vi "hpcnc visa write read.vi"(8 "error in (no error)":errorcluster, 10 "Send data":string, 11 "CNC COM in":refnum<visa-resource-name>) -> (0 "error out":errorcluster, 1 "Receive buffer":string, 2 "Receive count":u32, 3 "CNC COM out":refnum<visa-resource-name>)   [LabVIEW 2014, in "HPCNC.lvlib"]
uses:
  HPCNC.lvlib
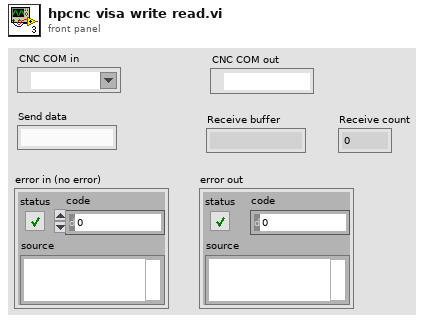
[diagram p1: front panel]
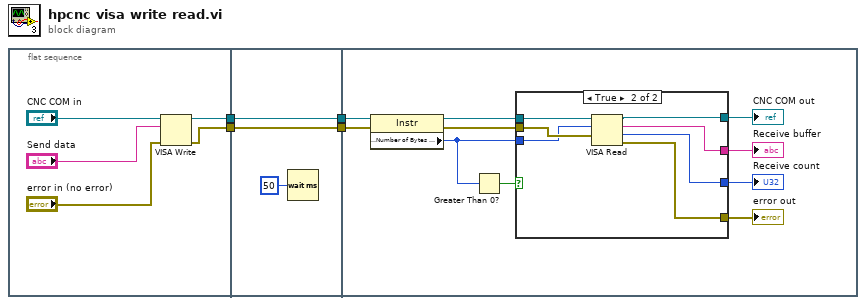
[diagram p0: block diagram]
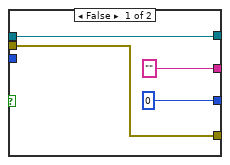
[diagram p2: hidden frame]
diagram:
  n1 = flat-sequence {
    tunnel: [w6] -> w3
    tunnel: [w5] -> w1
    tunnel: [w11] -> w4
    tunnel: w3 -> [w11]
    tunnel: [w10] -> w2
    tunnel: w1 -> [w10]
    tunnel: w4 -> [w14]
    tunnel: w2 -> [w13]
    frame #0 {
      n2 = VISA Write(VISA resource name="CNC COM in", write buffer="Send data", error in (no error)="error in (no error)") -> (VISA resource name out=w6:refnum<visa-resource-name>, error out=w5:errorcluster)  [unwired: 1 out]
    }
    frame #1 {
      n3 = Wait (ms)(milliseconds to wait=u32 50) -> ()  [unwired: 1 out]
    }
    frame #2 {
      n4 = property class="Instr"(reference=w14, error in=w13) -> (reference out=w16:refnum<visa-resource-name>, error out=w17:errorcluster, "Serial Settings:Number of Bytes at Serial Port"=w18:u32)
      n5 = Greater Than 0?(x=w18) -> (x > 0?=w15:bool)
      n6 = case shown="True" w15 {
        tunnel: w16 -> [w26 w33]
        tunnel: w17 -> [w23 w32]
        tunnel: w18 -> [_ w31]
        tunnel: [w26 w30] -> w19
        tunnel: ["" ("read buffer") w29] -> w20
        tunnel: [0 w28] -> w21
        tunnel: [w23 w27] -> w22
        frame False {
        }
        frame True {
          n7 = VISA Read(VISA resource name=w33, byte count=w31, error in (no error)=w32) -> (VISA resource name out=w30:refnum<visa-resource-name>, read buffer=w29:string, return count=w28:u32, error out=w27:errorcluster)
        }
      }
      "Receive buffer" <- w20
      "CNC COM out" <- w19
      "error out" <- w22
      "Receive count" <- w21
    }
  }
